vi "Write to HR DB_byRef.vi"(8 "error in (no error)":errorcluster, 9 "Values":u16[](array[numeric]), 10 "Modbus Address":u16, 11 "Cache Ref in":refnum<data-value>) -> (0 "error out":errorcluster, 3 "Cache Ref out":refnum<data-value>)   [LabVIEW 2018, in "MB PLC Client.lvlib" / "MB Data Block.lvclass"]
uses:
  MB Data Block.lvclass
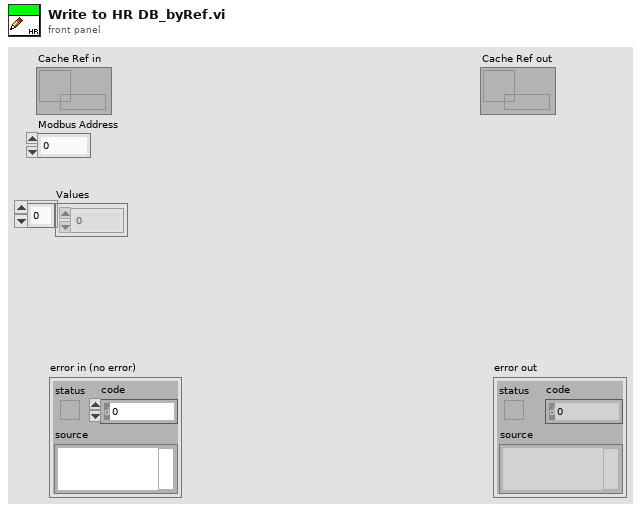
[diagram p1: front panel]
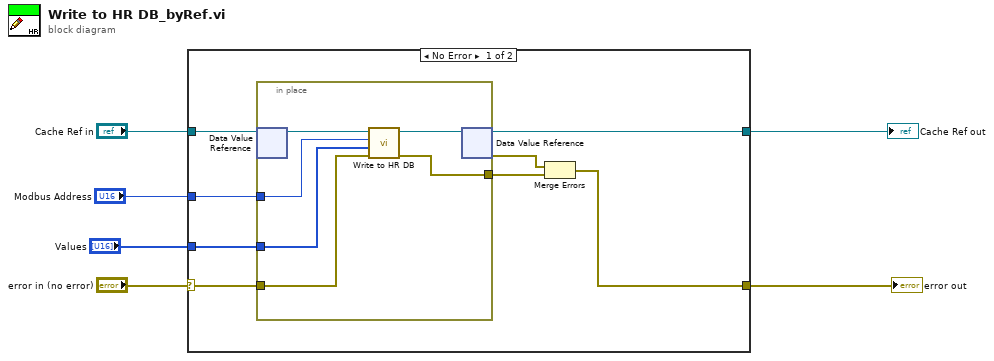
[diagram p0: block diagram]
diagram:
  n1 = case shown="No Error" "error in (no error)" {
    selector: "error in (no error)" -> [w7 w22]
    tunnel: "Cache Ref in" -> [w14 w21]
    tunnel: [w13 w21] -> w5
    tunnel: "Modbus Address" -> [w12 _]
    tunnel: "Values" -> [w11 _]
    tunnel: [w8 w22] -> w2
    frame No Error {
      n2 = in-place {
        in-place-border: w7 -> [w19]
        in-place-border: [w15] -> w10
        in-place-border: w12 -> [w17]
        in-place-border: w11 -> [w18]
        n3 = in-place-dvr #1(w14) -> (w20:refnum<class "MB Data Block.lvclass">)  [unwired: 1 out]
        n4 = call-dynamic "Write to HR DB.vi"("error in (no error)"=w19, "Values"=w18, "Modbus Address"=w17, "MB Cache in"=w20) -> ("error out"=w15:errorcluster, "MB Cache out"=w16:refnum<class "MB Data Block.lvclass">)  [unwired: 6 in]
        n5 = in-place-dvr #1(w16) -> (w13:refnum<data-value>, w9:errorcluster)
      }
      n6 = Merge Errors(w9, w10) -> (w8:errorcluster)
    }
    frame Error {
    }
  }
  "error out" <- w2
  "Cache Ref out" <- w5
